vi "drawe.vi"(8 "Ysize":i32, 9 "Xsize":i32, 11 "pos array":i32[][](array[numeric])) -> (2 "img out":i32[][](array[numeric]))   [LabVIEW 2020]
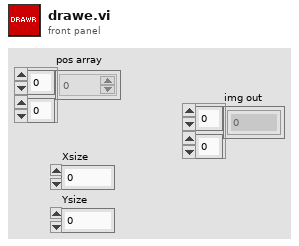
[diagram p1: front panel]
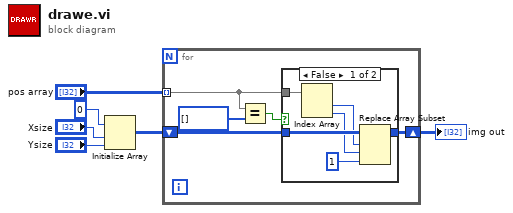
[diagram p0: block diagram]
diagram:
  n1 = Initialize Array(u16 0 ("element"), "Xsize", "Ysize") -> (w2:u16[][])
  n2 = for {
    tunnel: "pos array" -> [w9] mode=indexing
    shift-right: [w10] -> w6
    shift-left: w2 -> [w11]
    n3 = Equal?(x=w9, y=i32[] []) -> (x = y?=w7:bool)
    n4 = case shown="False" w7 {
      tunnel: w11 -> [w17 w18]
      tunnel: w9 -> [w16 _]
      tunnel: [w12 w18] -> w10
      frame False {
        n5 = Index Array(array=w16) -> (element #1=w15:i32, element #2=w14:i32)  [unwired: 2 in]
        n6 = Replace Array Subset(array=w17, new element=u32 1 ("new element/subarray"), index (row)=w15, index (col)=w14) -> (w12:u16[][])
      }
      frame True {
      }
    }
  }
  "img out" <- w6
